vi "Hardware - NI 9269-1 (Analog Output) Host.vi"() -> ()   [LabVIEW 2015, in "ECS-Host.lvlib"]
uses:
  ECS-Host.lvlib
  <vilib>/addons/Software Calibration Management/XControls/TBL1D.xctl
panel:
  out "FPGAWriteError":bool
  out "Ch3_TblOut":sgl caption="[]" format="%#.3g"
  in  "Ch3_Tbl":cluster{"X":sgl[], "Y":sgl[]}(xcontrol) caption="[]"
  in  "Ch3_Req":sgl caption="[]" format="%#.3g"
  out "Ch2_TblOut":sgl caption="[]" format="%#.3g"
  in  "Ch2_Tbl":cluster{"X":sgl[], "Y":sgl[]}(xcontrol) caption="[]"
  in  "Ch2_Req":sgl caption="[]" format="%#.3g"
  out "Ch1_TblOut":sgl caption="[]" format="%#.3g"
  in  "Ch1_Tbl":cluster{"X":sgl[], "Y":sgl[]}(xcontrol) caption="[]"
  in  "Ch1_Req":sgl caption="[]" format="%#.3g"
  out "Ch0_TblOut":sgl caption="[]" format="%#.3g"
  in  "Ch0_Req":sgl caption="[]" format="%#.3g"
  in  "Ch0_Tbl":cluster{"X":sgl[], "Y":sgl[]}(xcontrol) caption="[]"
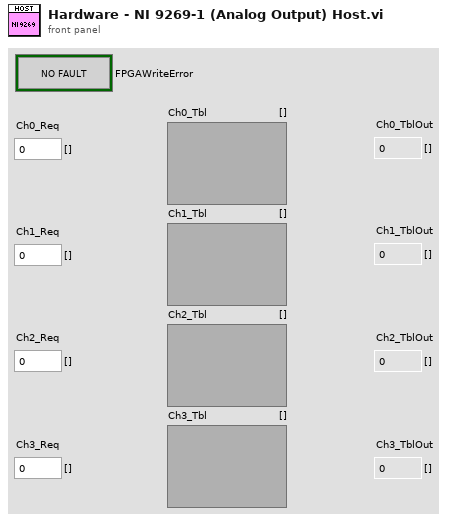
[diagram p1: front panel]
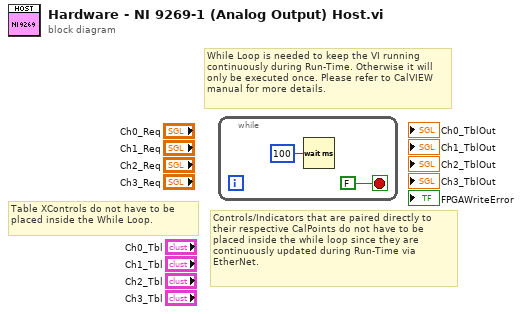
[diagram p0: block diagram]
diagram:
  # "Table XControls do not have to be placed inside the While Loop."
  # "Controls/Indicators that are paired directly to their respective CalPoints do not have to be placed inside the while loop since they are continuously updated during Run-Time via EtherNet."
  # "While Loop is needed to keep the VI running\ncontinuously during Run-Time. Otherwise it will only be executed once. Please refer to CalVIEW manual for more details."
  n1 = while {
    stop <- FALSE stop-if-true
    n2 = Wait (ms)(milliseconds to wait=u32 100) -> ()  [unwired: 1 out]
  }
